vi "set_delay_TRIG1.vi"(0 "VISA resource name":refnum<visa-resource-name>, 5 "error in":errorcluster, 6 "A ref":u32(slide) scale=0.0..3.0, 7 "A":dbl min=0.0 max=999.999999999995 format="%.12f", 8 "B ref":u32(slide) scale=0.0..3.0, 9 "B":dbl min=0.0 max=999.999999999995 format="%.12f", 10 "C ref":u32(slide) scale=0.0..3.0, 11 "C":dbl min=0.0 max=999.999999999995 format="%.12f", 12 "D ref":u32(slide) scale=0.0..3.0, 13 "D":dbl min=0.0 max=999.999999999995 format="%.12f") -> (14 "VISA resource name out":refnum<visa-resource-name>, 19 "error out":errorcluster)   [LabVIEW 2011]
doc: "This subVI sets the delay of the output channels relative to other channels or to the time reference T0 .\nControls A=, B= , C= and D= specify the reference channel and \nA, B, C, and D set the delay time in seconds .\nA Delay Linkage Error will be caused by an attempt to totally disconnect a time reference from T0 ."
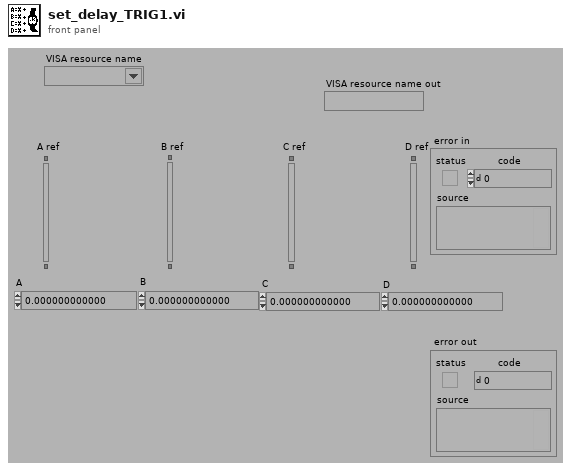
[diagram p1: front panel]
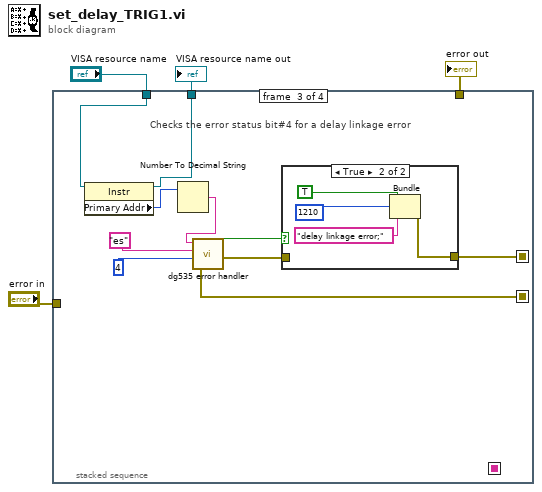
[diagram p0: block diagram]
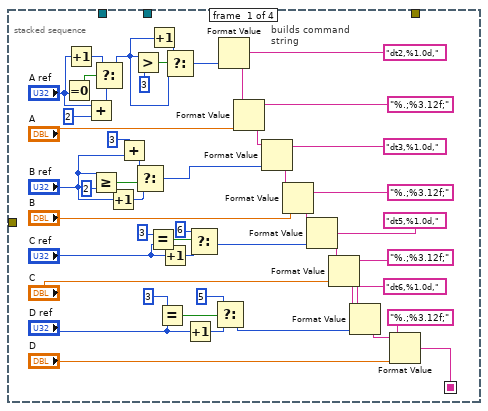
[diagram p2: hidden frame]
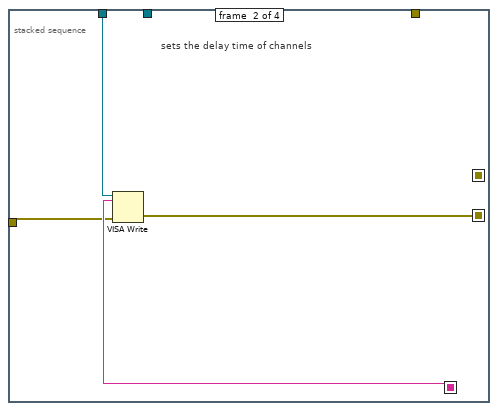
[diagram p3: hidden frame]
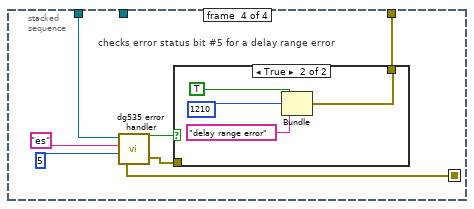
[diagram p5: hidden frame]
diagram:
  n1 = stacked-sequence {
    seq-local: [w35 _ _ _] -> [_ w57 _ _]
    seq-local: [_ w55 _ _] -> [_ _ w67 _]
    seq-local: [_ _ w64 _] -> [_ _ _ w73]
    tunnel: "VISA resource name" -> [_ w54 w61 w76]
    tunnel: "error in" -> [_ w56 _ _]
    tunnel: [_ _ _ w77] -> w3
    tunnel: [_ _ w58 _] -> w1
    frame #0 {
      # "builds command\nstring"
      n2 = Equal To 0?(x="A ref") -> (x = 0?=w16:bool)
      n3 = Increment(x="A ref") -> (x+1=w6:u32)
      n4 = Add(x="A ref", y=2) -> (x+y=w13:u32)
      n5 = Greater Or Equal?(x="B ref", y=2) -> (x >= y?=w19:bool)
      n6 = Select(t=w6, s=w16, f=w13) -> (s? t:f=w5:u32)
      n7 = Increment(x="B ref") -> (x+1=w17:u32)
      n8 = Add(x=3, y="B ref") -> (x+y=w20:u32)
      n9 = Greater?(x=w5, y=3) -> (0:w11:bool)
      n10 = Select(t=w20, s=w19, f=w17) -> (s? t:f=w18:u32)
      n11 = Equal?(x=3, y="C ref") -> (x = y?=w27:bool)
      n12 = Increment(x=w5) -> (x+1=w10:u32)
      n13 = Equal?(x=3, y="D ref") -> (x = y?=w32:bool)
      n14 = Increment(x="C ref") -> (x+1=w23:u32)
      n15 = Select(t=w10, s=w11, f=w5) -> (s? t:f=w9:u32)
      n16 = Increment(x="D ref") -> (x+1=w25:u32)
      n17 = Select(t=6, s=w27, f=w23) -> (s? t:f=w22:u32)
      n18 = Select(t=5, s=w32, f=w25) -> (s? t:f=w29:u32)
      n19 = Format Value(format string="dt2,%1.0d,", value (0)=w9) -> (output string=w46:string)  [unwired: 1 in]
      n20 = Format Value(string ("")=w46, format string="%.;%3.12f;", value (0)="A") -> (output string=w45:string)
      n21 = Format Value(string ("")=w45, format string="dt3,%1.0d,", value (0)=w18) -> (output string=w49:string)
      n22 = Format Value(string ("")=w49, format string="%.;%3.12f;", value (0)="B") -> (output string=w34:string)
      n23 = Format Value(string ("")=w34, format string="dt5,%1.0d,", value (0)=w22) -> (output string=w38:string)
      n24 = Format Value(string ("")=w38, format string="%.;%3.12f;", value (0)="C") -> (output string=w36:string)
      n25 = Format Value(string ("")=w36, format string="dt6,%1.0d,", value (0)=w29) -> (output string=w43:string)
      n26 = Format Value(string ("")=w43, format string="%.;%3.12f;", value (0)="D") -> (output string=w35:string)
    }
    frame #1 {
      # "sets the delay time of channels"
      n27 = VISA Write(VISA resource name=w54, write buffer=w57, error in (no error)=w56) -> (error out=w55:errorcluster)  [unwired: 2 out]
    }
    frame #2 {
      # "Checks the error status bit#4 for a delay linkage error"
      n28 = property class="Instr"(reference=w61) -> (reference out=w58:refnum<visa-resource-name>, "Primary Addr"=w60:u16)  [unwired: 1 in, 1 out]
      n29 = Number To Decimal String(number=w60) -> (decimal integer string=w59:string)  [unwired: 1 in]
      n30 = call "dg535 error handler.vi"("error in"=w67, "check bit #"=4, "command string"="es", "GPIB address"=w59) -> ("error out"=w65:errorcluster, "error found"=w66:bool)
      n31 = case shown="True" w66 {
        tunnel: w65 -> [w68 _]
        tunnel: [w68 w69] -> w64
        frame False {
        }
        frame True {
          n32 = Bundle(TRUE, 1210, "delay linkage error;") -> (w69:errorcluster)  [unwired: 1 in]
        }
      }
    }
    frame #3 {
      # "checks error status bit #5 for a delay range error"
      n33 = call "dg535 error handler.vi"("error in"=w73, "check bit #"=5, "command string"="es", "GPIB address"=w76) -> ("error out"=w78:errorcluster, "error found"=w79:bool)
      n34 = case shown="True" w79 {
        tunnel: w78 -> [w80 _]
        tunnel: [w80 w81] -> w77
        frame False {
        }
        frame True {
          n35 = Bundle(TRUE, 1210, "delay range error") -> (w81:errorcluster)  [unwired: 1 in]
        }
      }
    }
  }
  "error out" <- w3
  "VISA resource name out" <- w1
